vi "WriteVirtualSelect.vi"(8 "error in (no error)":errorcluster, 10 "VirtualSelectIdx":i32, 11 "Project.lvclass In":refnum<class "Project.lvclass">) -> (0 "error out":errorcluster, 3 "Project.lvclass Out":refnum<class "Project.lvclass">)   [LabVIEW 2014, in "Project.lvclass"]
uses:
  Project.lvclass
  Project.lvclass/Project.ctl
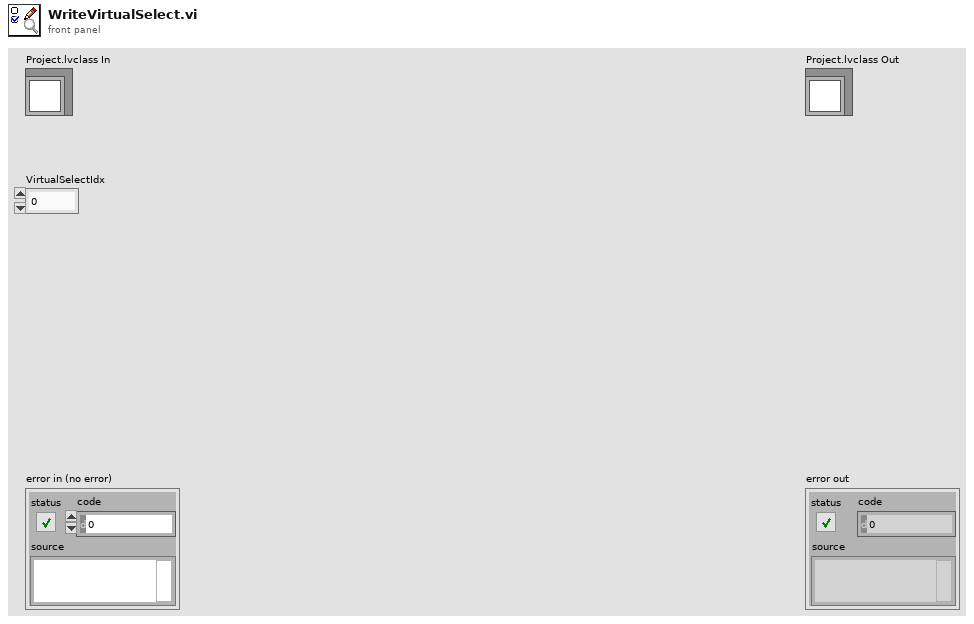
[diagram p1: front panel]
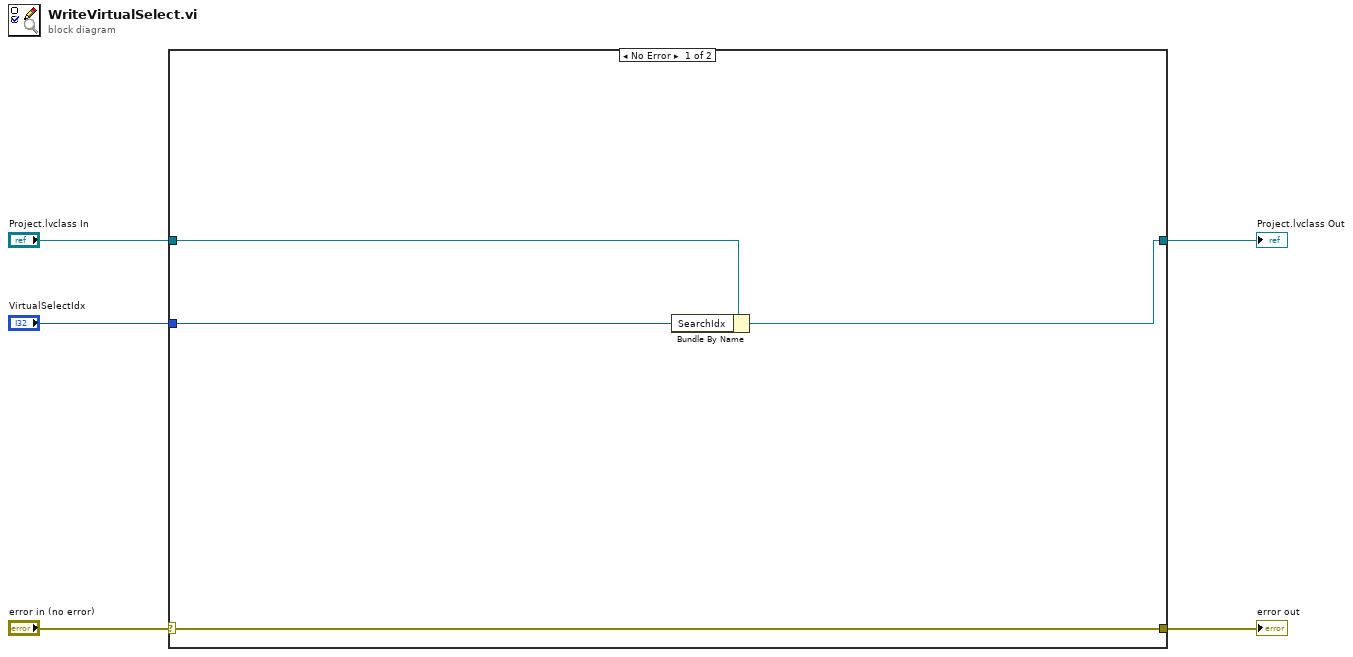
[diagram p0: block diagram]
diagram:
  n1 = case shown="No Error" "error in (no error)" {
    selector: "error in (no error)" -> [w9 w11]
    tunnel: [w9 w11] -> w4
    tunnel: "Project.lvclass In" -> [w8 w10]
    tunnel: "VirtualSelectIdx" -> [w7 _]
    tunnel: [w6 w10] -> w1
    frame No Error {
      n2 = Bundle By Name(cluster=w8, "SearchIdx"=w7) -> (w6:refnum<class "Project.lvclass">)
    }
    frame Error {
    }
  }
  "error out" <- w4
  "Project.lvclass Out" <- w1
